vi "Read Two Flukes.vi"() -> ()   [LabVIEW 2012]
uses:
  <vilib>/Utility/file.llb/Write To Spreadsheet File (DBL).vi
panel:
  in  "Save Data?":bool=TRUE
  out "Currrent Point":cluster{"x value":dbl, "y value":dbl} {"y value" format="%^.6e"; "x value" format="%^.6e"}
  in  "stop":bool
  out "XY Graph":cluster{"X":dbl, "Y":dbl}[](graph)
  out "y unit":string
  out "x unit":string
  in  "VISA resource name y":refnum<visa-resource-name>="GPIB0::15::INSTR"
  in  "VISA resource name x":refnum<visa-resource-name>="GPIB0::14::INSTR"
  in  "error in":errorcluster
  out "error out":errorcluster
  in  "trigger mode y":u16(ring) items=["internal - continuous trigger", "external - rear panel trigger with delay", "external - bus trigger with delay", "external - rear panel trigger", "external - bus trigger"]
  in  "trigger mode x":u16(ring) items=["internal - continuous trigger", "external - rear panel trigger with delay", "external - bus trigger with delay", "external - rear panel trigger", "external - bus trigger"]
  in  "Dwell Time (ms)":i32=50
  out "AutoRange y":bool
  in  "rate set y":u16(ring) items=["slow", "medium", "fast"]
  in  "range set y":u16(ring)=6 items=["autorange", "200mV, 200 ohms", "2V, 2 kohms", "20V, 20 kohms", "200V, 200 kohms", "1000Vdc, 700 Vac, 2 Mohms", "20 Mohms"]
  in  "function set y":u16(ring) items=["volts DC", "volts AC", "2-wire k.ohms", "4-wire k.ohms", "mA DC", "mA AC"]
  out "AutoRange x":bool
  in  "rate set x":u16(ring) items=["slow", "medium", "fast"]
  in  "range set x":u16(ring)=6 items=["autorange", "200mV, 200 ohms", "2V, 2 kohms", "20V, 20 kohms", "200V, 200 kohms", "1000Vdc, 700 Vac, 2 Mohms", "20 Mohms"]
  in  "function set x":u16(ring) items=["volts DC", "volts AC", "2-wire k.ohms", "4-wire k.ohms", "mA DC", "mA AC"]
  # "Y AXIS"
  # "X AXIS"
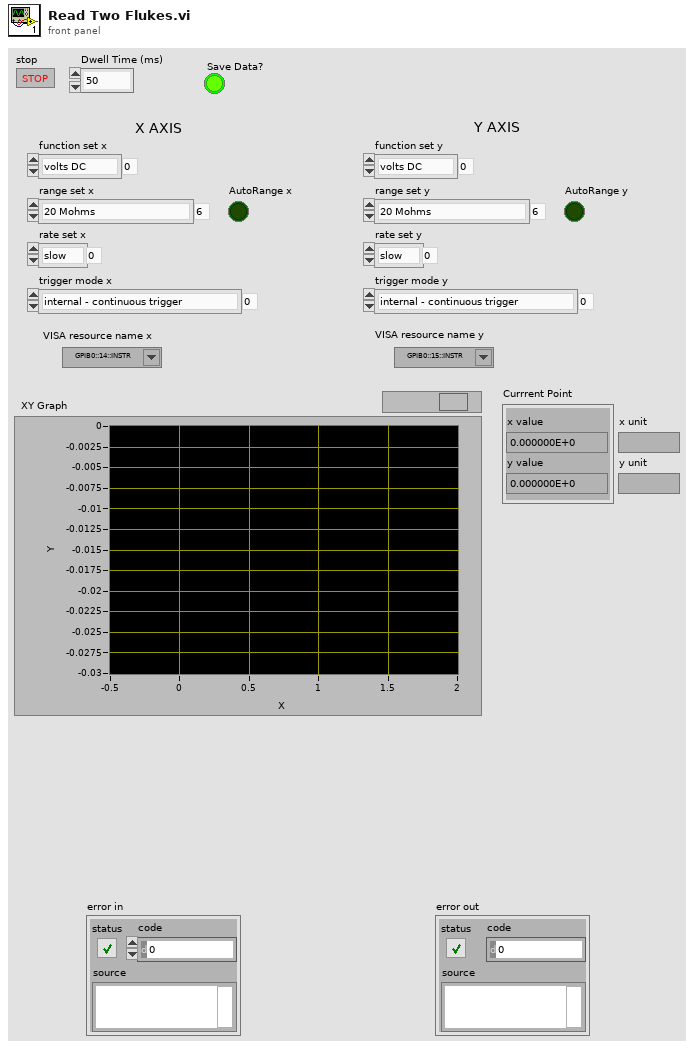
[diagram p1: front panel]
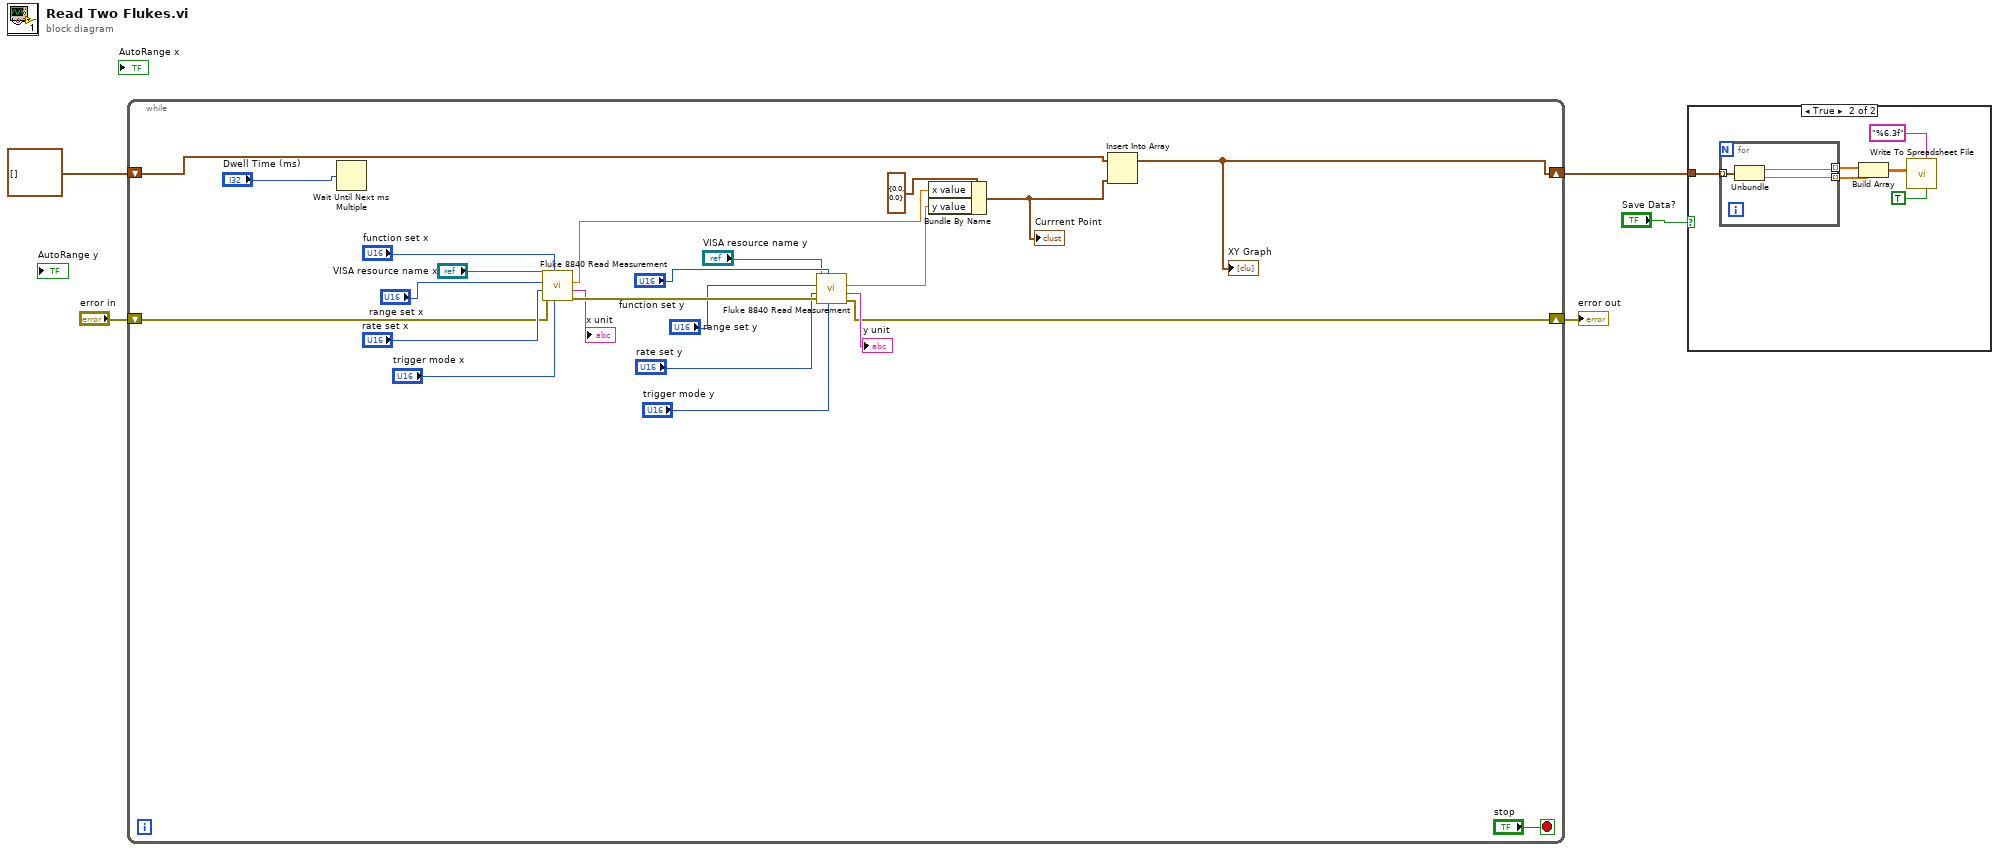
[diagram p0: block diagram]
diagram:
  n1 = while {
    shift-right: [w15] -> w5
    shift-left: "error in" -> [w14]
    shift-right: [w6] -> w1
    shift-left: cluster{"X":dbl, "Y":dbl}[] [] ("XY Graph") -> [w11]
    stop <- "stop" stop-if-true
    n2 = Wait Until Next ms Multiple(millisecond multiple="Dwell Time (ms)") -> ()  [unwired: 1 out]
    n3 = call "Fluke 8840 Read Measurement.vi"("trigger mode (0:internal)"="trigger mode x", "function (0:volts DC)"="function set x", "error in (no error)"=w14, "rate (0:slow)"="rate set x", "range (0:auto)"="range set x", "VISA resource name"="VISA resource name x") -> ("error out"=w26:errorcluster, "unit"=→"x unit":string, "measurement"=w9:dbl)  [unwired: 3 out]
    n4 = call "Fluke 8840 Read Measurement.vi"("trigger mode (0:internal)"="trigger mode y", "function (0:volts DC)"="function set y", "error in (no error)"=w26, "rate (0:slow)"="rate set y", "range (0:auto)"="range set y", "VISA resource name"="VISA resource name y") -> ("error out"=w15:errorcluster, "unit"=→"y unit":string, "measurement"=w8:dbl)  [unwired: 3 out]
    n5 = Bundle By Name(cluster=cluster{"x value":dbl, "y value":dbl} {"x value"=0.0, "y value"=0.0} ("Currrent Point"), "x value"=w9, "y value"=w8) -> (w7:cluster{"x value":dbl, "y value":dbl})
    "Currrent Point" <- w7
    n6 = Insert Into Array(array=w11, new element=w7) -> (w6:cluster{"X":dbl, "Y":dbl}[])  [unwired: 1 in]
    "XY Graph" <- w6
  }
  "error out" <- w5
  n7 = case shown="True" "Save Data?" {
    tunnel: w1 -> [_ w34]
    frame False {
    }
    frame True {
      n8 = for {
        tunnel: w34 -> [w37] mode=indexing
        tunnel: [w36] -> w32 mode=indexing
        tunnel: [w35] -> w33 mode=indexing
        n9 = Unbundle(w37) -> ("X"=w35:dbl, "Y"=w36:dbl)
      }
      n10 = Build Array(w33, w32) -> (w31:dbl[][])
      n11 = call-poly <vilib>:"Write To Spreadsheet File.vi"("transpose? (no:F)"=TRUE, "format (%.3f)"="%6.3f", "2D data"=w31) -> ()  [unwired: 5 in, 1 out]
    }
  }
